vi "Node Contants.vi"(8 "error in (no error)":errorcluster, 11 "Node Value in":refnum<class "Node Value.lvclass">) -> (0 "error out":errorcluster, 2 "Constants":T1, 3 "Node Value out":refnum<class "Node Value.lvclass">)   [LabVIEW 2019, in "Node Value.lvclass"]
uses:
  Node Value.lvclass
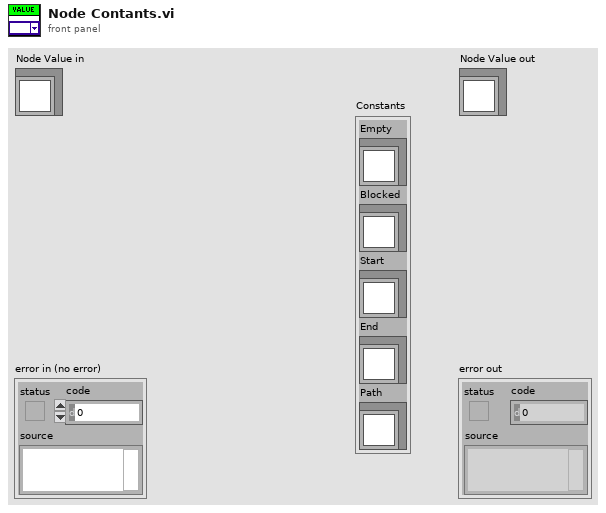
[diagram p1: front panel]
types:
  T1 = cluster{"Empty":refnum<class "Node Value.lvclass">, "Blocked":refnum<class "Node Value.lvclass">, "Start":refnum<class "Node Value.lvclass">, "End":refnum<class "Node Value.lvclass">, "Path":refnum<class "Node Value.lvclass">}
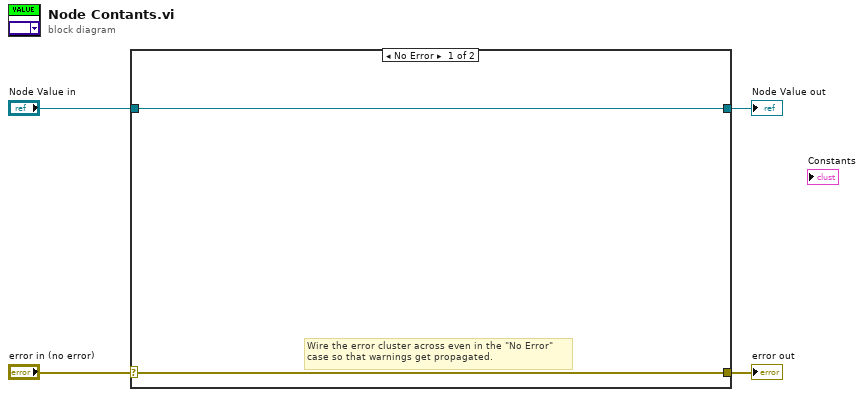
[diagram p0: block diagram]
diagram:
  n1 = case shown="No Error" "error in (no error)" {
    selector: "error in (no error)" -> [w5 w8]
    tunnel: [w5 w8] -> w3
    tunnel: [w6 w7] -> w1
    tunnel: "Node Value in" -> [w6 w7]
    frame No Error {
      # "Wire the error cluster across even in the \"No Error\"\ncase so that warnings get propagated."
    }
    frame Error {
    }
  }
  "error out" <- w3
  "Node Value out" <- w1
